vi "Read Data.vi"(8 "error in (no error)":errorcluster, 9 "timeout in ms (-1)":i32=-1) -> (0 "error out":errorcluster, 1 "timed out?":bool, 2 "Monitor Data":refnum<class "Monitor Data.lvclass">)   [LabVIEW 2017, in "Debug Monitor.lvclass"]
uses:
  Debug Monitor.lvclass
  Source/Monitor Data/Monitor Data.lvclass
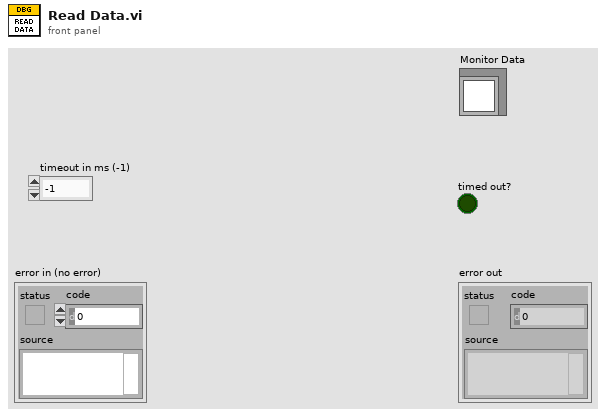
[diagram p1: front panel]
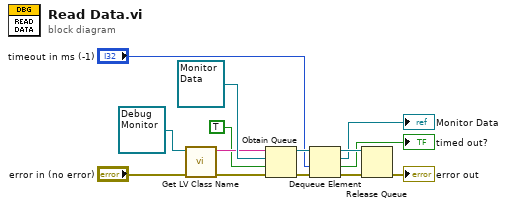
[diagram p0: block diagram]
diagram:
  n1 = call <vilib>:"Get LV Class Name.vi"("error in (no error)"="error in (no error)", "object"=refnum<class "Debug Monitor.lvclass"> refnum ("Actor out")) -> ("error out"=w12:errorcluster, "class name"=w13:string)  [unwired: 8 in]
  n2 = Obtain Queue(name (unnamed)=w13, element data type=refnum<class "Monitor Data.lvclass"> refnum ("Monitor Data"), create if not found? (T)=TRUE, error in (no error)=w12) -> (queue out=w8:refnum<queue>, error out=w7:errorcluster)  [unwired: 1 in, 1 out]
  n3 = Dequeue Element(queue=w8, timeout in ms (-1)="timeout in ms (-1)", error in (no error)=w7) -> (queue out=w6:refnum<queue>, element=→"Monitor Data":refnum<class "Monitor Data.lvclass">, timed out?=→"timed out?":bool, error out=w5:errorcluster)
  n4 = Release Queue(queue=w6, error in (no error)=w5) -> (error out=→"error out":errorcluster)  [unwired: 1 in, 2 out]
